vi "move_backlash_loop.vi"(6 "Axis enable":bool[](array[boolean])=[TRUE, TRUE, TRUE, TRUE], 7 "Trio handle":refnum<k7>, 8 "error in":errorcluster, 9 "Axis positions":dbl[](array[numeric]), 11 "Absolute":bool=TRUE) -> (0 "error out":errorcluster, 1 "Final axis errors":i32[](array[numeric]))   [LabVIEW 2024]
panel:
  out "Retry count":i32
  in  "Max error":i32=3
  # "Loop doing backlash move until the error is small enough."
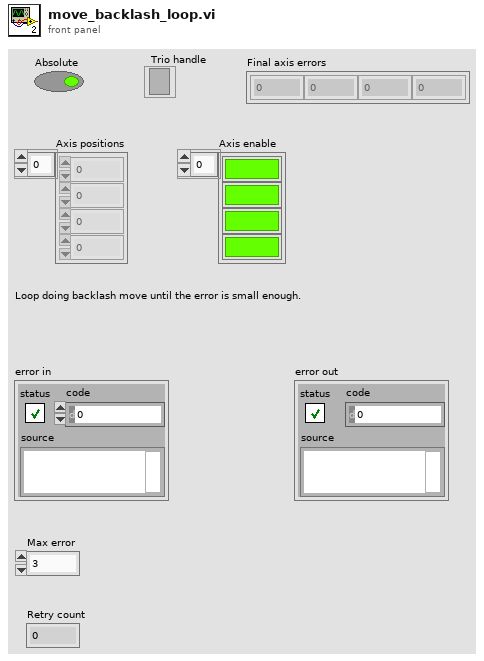
[diagram p1: front panel]
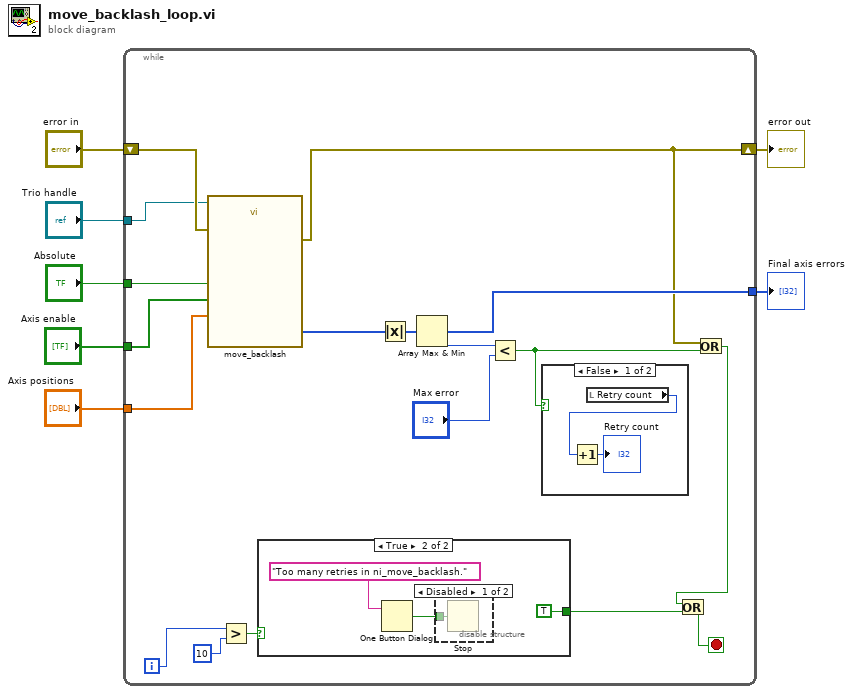
[diagram p0: block diagram]
diagram:
  n1 = while {
    tunnel: "Absolute" -> [w24]
    tunnel: "Axis positions" -> [w23]
    tunnel: "Axis enable" -> [w22]
    tunnel: [w14] -> w2
    shift-right: [w12] -> w3
    shift-left: "error in" -> [w21]
    tunnel: "Trio handle" -> [w13]
    i -> [w17]
    stop <- w8 stop-if-true
    n2 = call "move_backlash.vi"("Axis enable"=w22, "error in"=w21, "Axis positions"=w23, "Absolute"=w24, "Trio handle"=w13) -> ("error out"=w12:errorcluster, "Final axis errors"=w14:i32[])  [unwired: 5 in]
    n3 = Greater?(x=w17, y=10) -> (0:w15:bool)
    n4 = case shown="True" w15 {
      tunnel: [_ TRUE ("x .or. y?")] -> w10
      frame False {
      }
      frame True {
        n5 = One Button Dialog(message="Too many retries in ni_move_backlash.") -> (true=w28:bool)  [unwired: 1 in]
        n6 = disable-structure shown="Disabled" {
          disable-tunnel: w28 -> [w30 _]
          frame Disabled {
            n7 = Stop(stop? (T)=w30) -> ()
          }
          frame Enabled {
          }
        }
      }
    }
    n8 = Absolute Value(x=w14) -> (abs(x)=w20:i32[])
    n9 = Array Max & Min(array=w20) -> (max value=w19:i32)  [unwired: 3 out]
    n10 = Less?(x=w19, y="Max error") -> (x < y?=w11:bool)
    n11 = case shown="False" w11 {
      frame False {
        n12 = local read "Retry count"() -> (w25:i32)
        n13 = Increment(x=w25) -> (x+1=→"Retry count":i32)
      }
      frame True {
      }
    }
    n14 = Or(x=w12, y=w11) -> (x .or. y?=w9:bool)
    n15 = Or(x=w9, y=w10) -> (x .or. y?=w8:bool)
  }
  "error out" <- w3
  "Final axis errors" <- w2
